vi "FTW-Message-Request-Reply.vi"(8 "FTW: Reply Error":errorcluster caption="error in", 11 "FTW Incoming Request":refnum<class "FTW-Message-HttpRequest.lvclass">) -> (0 "error out":errorcluster, 2 "Timed out?":bool)   [LabVIEW 2015, in "FTW-Message-HttpRequest.lvclass"]
uses:
  FTW-Message-HttpRequest.lvclass
  Endpoint/FTW-Endpoint.lvclass
panel:
  # "Inputs"
  # "Outputs"
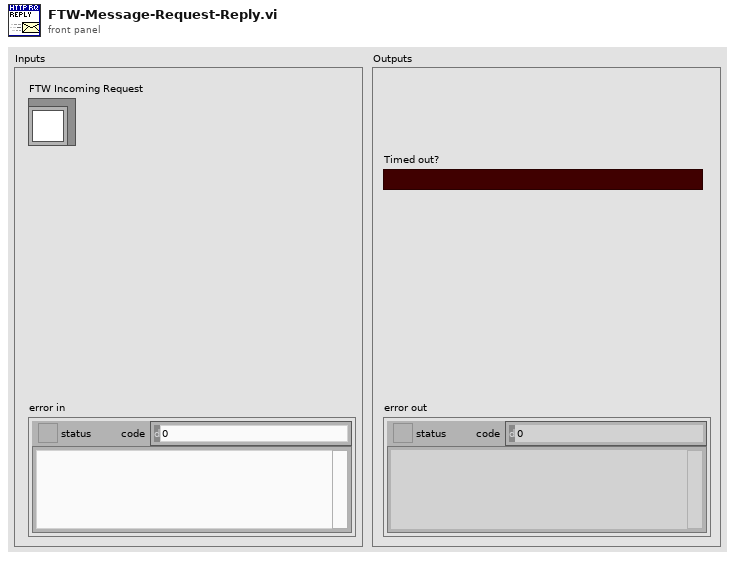
[diagram p1: front panel]
types:
  T1 = typedef "FTW-MessagePayload.ctl" = cluster{"Header":string, "Body":string, "FTW: Sender Identity":string, "FTW: Reply Address":string, "FTW: Reply Error":errorcluster}
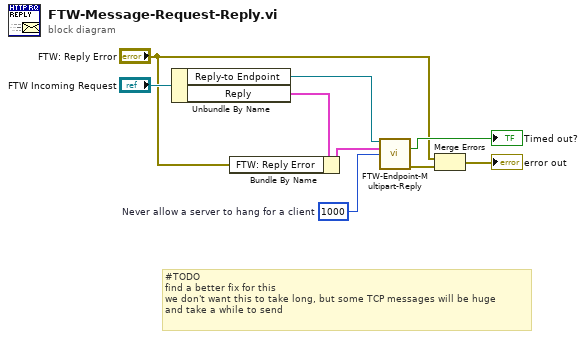
[diagram p0: block diagram]
diagram:
  w6 = 1000  # Never allow a server to hang for a client
  # "#TODO\nfind a better fix for this\nwe don't want this to take long, but some TCP messages will be huge\nand take a while to send"
  n1 = Unbundle By Name("FTW Incoming Request") -> ("Reply-to Endpoint"=w8:refnum<class "FTW-Endpoint.lvclass">, "Reply"=w3:T1)
  n2 = Bundle By Name(cluster=w3, "FTW: Reply Error"="FTW: Reply Error") -> (w2:T1)
  n3 = call-dynamic "FTW-Endpoint-Multipart-Reply.vi"("FTW Endpoint"=w8, "Message"=w2, "Timeout"=w6) -> ("Timed out?"=→"Timed out?":bool, "error out"=w7:errorcluster)  [unwired: 10 in, 1 out]
  n4 = Merge Errors("FTW: Reply Error", w7) -> (→"error out":errorcluster)
